vi "Destroy.vi"(0 "scripts manager in":refnum<class "scripts manager.lvclass">, 11 "error in (no error)":errorcluster) -> (4 "scripts manager out":refnum<class "scripts manager.lvclass">, 15 "error out":errorcluster)   [LabVIEW 2016, in "scripts manager.lvclass"]
uses:
  scripts manager.lvclass
  functions/functionsbase/functionbase.lvclass
  common/Line Details.ctl
  scripts manager.lvclass/scripts manager.ctl
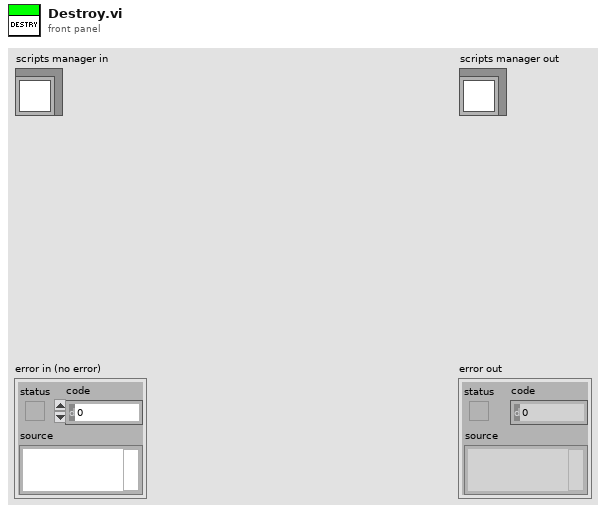
[diagram p1: front panel]
types:
  T1 = typedef "Line Details.ctl" = cluster{"Line#":i64, "Indent#":i64, "Function":string}
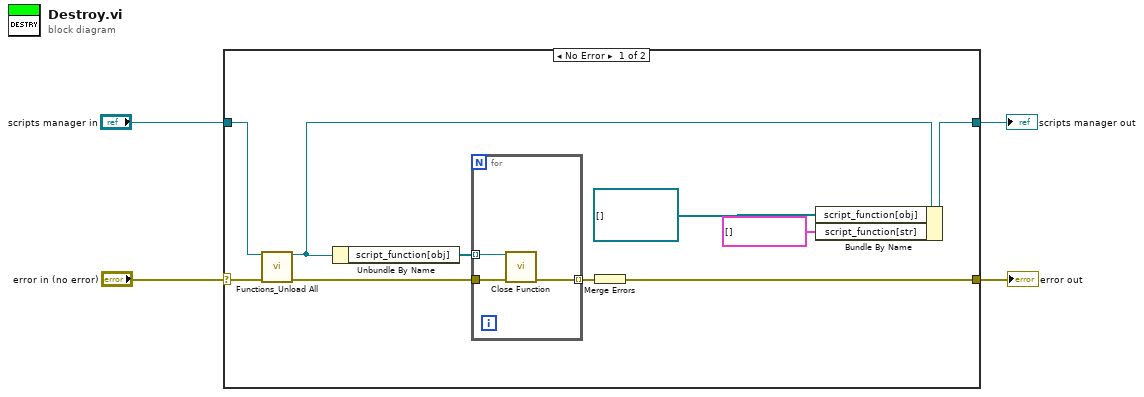
[diagram p0: block diagram]
diagram:
  n1 = case shown="No Error" "error in (no error)" {
    selector: "error in (no error)" -> [w14 w19]
    tunnel: [w9 w19] -> w3
    tunnel: [w7 w18] -> w1
    tunnel: "scripts manager in" -> [w13 w18]
    frame No Error {
      n2 = call-dynamic "Functions_Unload All.vi"("scripts manager in"=w13, "error in (no error)"=w14) -> ("scripts manager out"=w8:refnum<class "scripts manager.lvclass">, "error out"=w11:errorcluster)  [unwired: 12 in]
      n3 = Unbundle By Name(w8) -> ("script_function[obj]"=w12:refnum<class "functionbase.lvclass">[])
      n4 = for {
        tunnel: w12 -> [w17] mode=indexing
        tunnel: w11 -> [w16]
        tunnel: [w15] -> w10 mode=indexing
        n5 = call-dynamic "Close Function.vi"("functionbase in"=w17, "error in (no error)"=w16) -> ("error out"=w15:errorcluster)  [unwired: 12 in, 1 out]
      }
      n6 = Merge Errors(w10) -> (w9:errorcluster)
      n7 = Bundle By Name(cluster=w8, "script_function[obj]"=refnum<class "functionbase.lvclass">[] [], "script_function[str]"=T1[] []) -> (w7:refnum<class "scripts manager.lvclass">)
    }
    frame Error {
    }
  }
  "error out" <- w3
  "scripts manager out" <- w1
